vi "globle_var.vi"() -> ()   [LabVIEW 2020]
panel:
  out "value":dbl
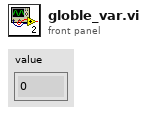
[diagram p1: front panel]
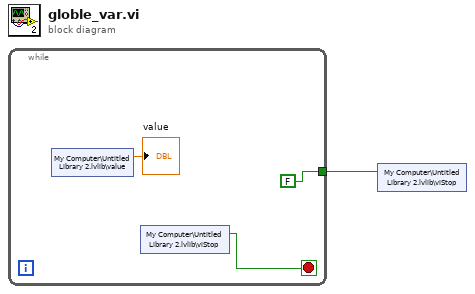
[diagram p0: block diagram]
diagram:
  n1 = while {
    tunnel: [FALSE] -> w1
    stop <- w3 stop-if-true
    n2 = shared-variable "My Computer\\Untitled Library 2.lvlib\\value"() -> (→"value":dbl)  [unwired: 1 in, 1 out]
    n3 = shared-variable "My Computer\\Untitled Library 2.lvlib\\viStop"() -> (w3:bool)  [unwired: 1 in, 1 out]
  }
  n4 = shared-variable "My Computer\\Untitled Library 2.lvlib\\viStop"(w1) -> ()  [unwired: 1 in, 1 out]
